vi "RegisterSettings.vi"(8 "error in":errorcluster, 11 "MainFGV_data":T1) -> (0 "error out":errorcluster, 3 "MainFGV_data out":T1)   [LabVIEW 2016]
uses:
  MainFGV_data.ctl
  Settings/config_board.ctl
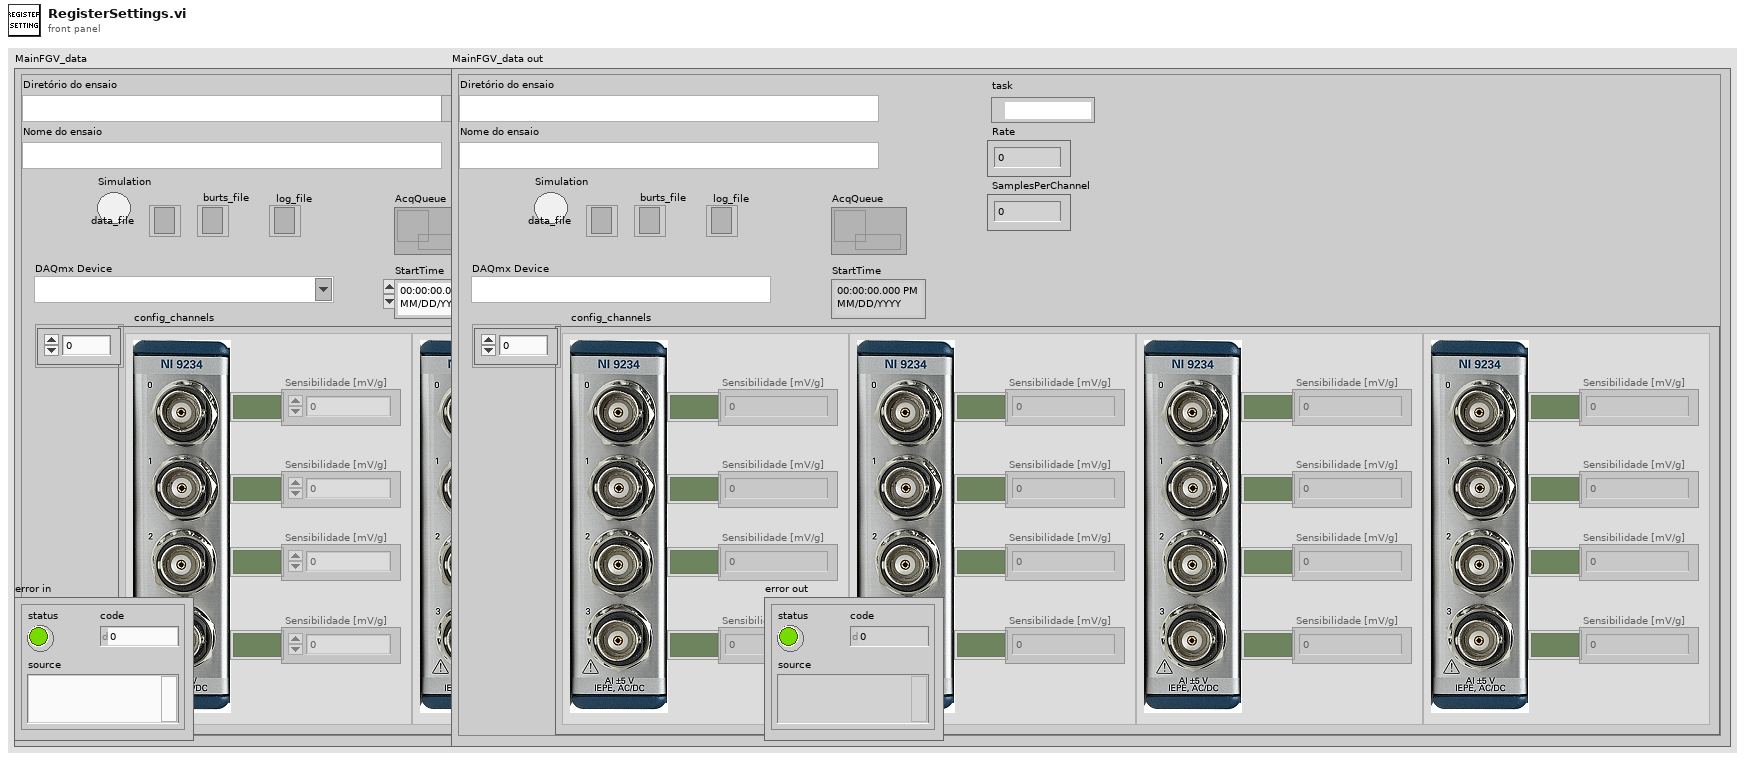
[diagram p1: front panel]
types:
  T1 = typedef "MainFGV_data.ctl" = cluster{"TestDir":path, "TestName":string, "Simulation":bool, "task":refnum<k21>, "data_file":refnum<file>, "burts_file":refnum<file>, "log_file":refnum<file>, "Rate":dbl, "SamplesPerChannel":dbl, "AcqQueue":refnum<queue>, "StartTime":timestamp, "config_channels":T2[], "DAQmx Device":tag}
  T2 = typedef "config_board.ctl" = cluster{"Sens0":dbl, "Active0":bool, "Sens1":dbl, "Active1":bool, "Sens2":dbl, "Active2":bool, "Sens3":dbl, "Active3":bool}
  T3 = enum16{"open", "replace", "create", "open or create", "replace or create", "replace or create with confirmation"}
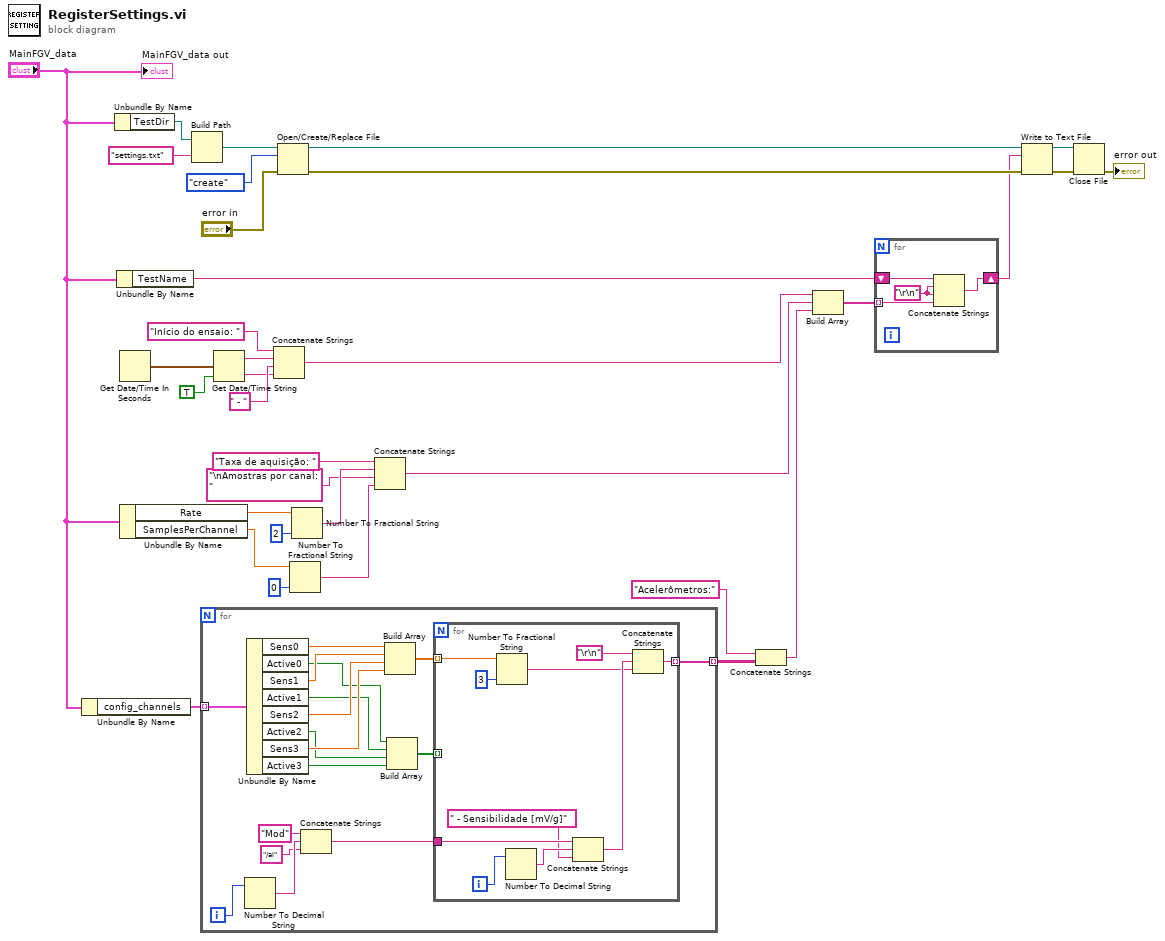
[diagram p0: block diagram]
diagram:
  n1 = Unbundle By Name("MainFGV_data") -> ("config_channels"=w17:T2[])
  n2 = Unbundle By Name("MainFGV_data") -> ("TestDir"=w34:path)
  n3 = Unbundle By Name("MainFGV_data") -> ("TestName"=w2:string)
  n4 = Get Date/Time In Seconds() -> (seconds since 1Jan1904=w1:timestamp)
  n5 = Unbundle By Name("MainFGV_data") -> ("Rate"=w24:dbl, "SamplesPerChannel"=w20:dbl)
  n6 = Build Path(base path=w34, name or relative path="settings.txt") -> (appended path=w32:path)
  n7 = for {
    tunnel: w17 -> [w50] mode=indexing
    tunnel: [w35] -> w16 mode=indexing
    i -> [w51]
    n8 = Number To Decimal String(number=w51) -> (decimal integer string=w39:string)  [unwired: 1 in]
    n9 = Unbundle By Name(w50) -> ("Sens0"=w49:dbl, "Active0"=w42:bool, "Sens1"=w48:dbl, "Active1"=w43:bool, "Sens2"=w47:dbl, "Active2"=w44:bool, "Sens3"=w46:dbl, "Active3"=w45:bool)
    n10 = Concatenate Strings("Mod" ("string"), w39, "/ai" ("string")) -> (w36:string)
    n11 = Build Array(w49, w48, w47, w46) -> (w40:dbl[])
    n12 = Build Array(w42, w43, w44, w45) -> (w41:bool[])
    n13 = for {
      tunnel: w41 -> [_] mode=indexing
      tunnel: w40 -> [w57] mode=indexing
      tunnel: w36 -> [w60]
      tunnel: [w52] -> w35 mode=indexing
      i -> [w61]
      n14 = Number To Fractional String(number=w57, precision (6)=i16 3) -> (F-format string=w54:string)  [unwired: 2 in]
      n15 = Number To Decimal String(number=w61) -> (decimal integer string=w59:string)  [unwired: 1 in]
      n16 = Concatenate Strings(w60, w59, " - Sensibilidade [mV/g]" ("string")) -> (w55:string)
      n17 = Concatenate Strings("\r\n", w55, w54) -> (w52:string)
    }
  }
  n18 = Get Date/Time String(seconds (now)=w1, want seconds? (F)=TRUE) -> (date string=w27:string, time string=w26:string)  [unwired: 1 in]
  n19 = Concatenate Strings("Início do ensaio: " ("string"), w27, " - " ("string"), w26) -> (w13:string)
  n20 = Open/Create/Replace File(file path (use dialog)=w32, error in="error in", operation (0:open)=T3."create") -> (refnum out=w6:refnum<file>, error out=w8:errorcluster)  [unwired: 3 in, 1 out]
  n21 = Number To Fractional String(number=w20, precision (6)=i16 0) -> (F-format string=w18:string)  [unwired: 2 in]
  n22 = Number To Fractional String(number=w24, precision (6)=i16 2) -> (F-format string=w22:string)  [unwired: 2 in]
  n23 = Concatenate Strings("Taxa de aquisição: " ("string"), w22, "\nAmostras por canal: " ("string"), w18) -> (w12:string)
  n24 = Concatenate Strings("Acelerômetros:" ("string"), w16) -> (w11:string)
  n25 = Build Array(w13, w12, w11) -> (w10:string[])
  n26 = for {
    tunnel: w10 -> [w64] mode=indexing
    shift-right: [w62] -> w7
    shift-left: w2 -> [w65]
    w63 = "\r\n"
    n27 = Concatenate Strings(w65, w63, w63, w64) -> (w62:string)
  }
  n28 = Write to Text File(file (use dialog)=w6, text=w7, error in=w8) -> (refnum out=w4:refnum<file>, error out=w5:errorcluster)  [unwired: 1 in, 1 out]
  n29 = Close File(refnum=w4, error in=w5) -> (error out=→"error out":errorcluster)  [unwired: 1 out]
  "MainFGV_data out" <- "MainFGV_data"
